vi "sub_conv_enc_v2.vi"(8 "code type":T1(ring)=enum."r=1/2 (13,17)", 11 "bitstream":i32[](array[numeric])) -> (3 "coded bits":i16[](array[numeric]))   [LabVIEW 2014]
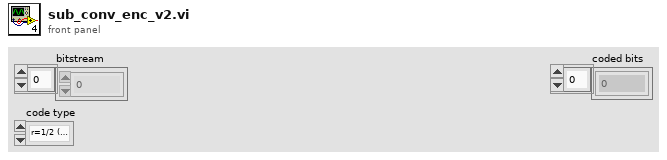
[diagram p1: front panel]
types:
  T1 = enum16{"r=1/2 (5,7)", "r=1/2 (13,17)", "r=1/4 (25,27,33,37)"}
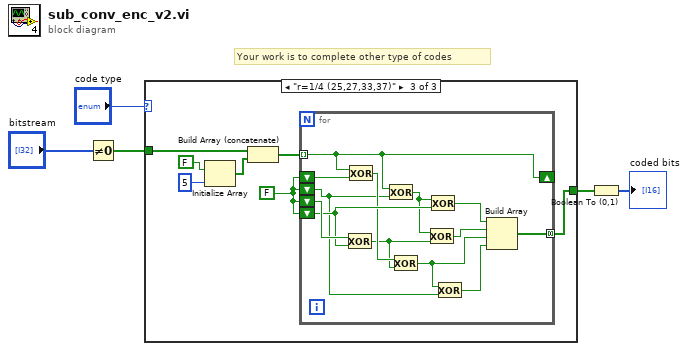
[diagram p0: block diagram]
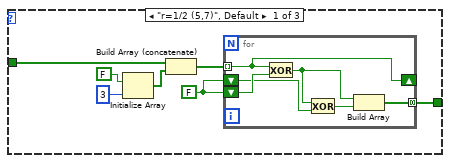
[diagram p2: hidden frame]
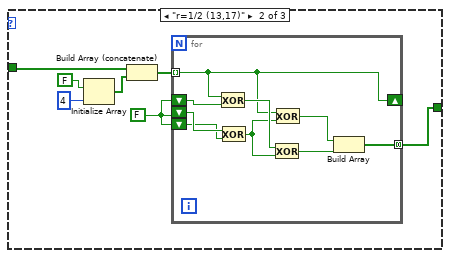
[diagram p3: hidden frame]
diagram:
  # "Your work is to complete other type of codes"
  n1 = Not Equal To 0?(x="bitstream") -> (x != 0?=w3:bool[])
  n2 = case shown="\"r=1/4 (25,27,33,37)\"" "code type" {
    tunnel: w3 -> [w8 w22 w38]
    tunnel: [w11 w20 w36] -> w2
    frame "r=1/2 (5,7)", Default {
      w12 = FALSE
      n3 = Initialize Array(FALSE, 3 ("dimension size")) -> (w7:bool[])
      n4 = Build Array (concatenate)(w8, w7) -> (w6:bool[])
      n5 = for {
        tunnel: w6 -> [w13] mode=indexing
        shift-right: [w13] -> _
        shift-left: w12 -> [w15]
        shift-left: w12 -> [w17]
        tunnel: [w18] -> w11 mode=concatenating
        n6 = Exclusive Or(1:w17, 2:w13) -> (0:w16:bool)
        n7 = Exclusive Or(1:w15, 2:w16) -> (0:w14:bool)
        n8 = Build Array(w16, w14) -> (w18:bool[])
      }
    }
    frame "r=1/2 (13,17)" {
      w19 = FALSE
      n9 = Initialize Array(FALSE, 4 ("dimension size")) -> (w23:bool[])
      n10 = Build Array (concatenate)(w22, w23) -> (w21:bool[])
      n11 = for {
        shift-right: [w29] -> _
        shift-left: w19 -> [w32]
        tunnel: w21 -> [w29] mode=indexing
        shift-left: w19 -> [w34]
        shift-left: w19 -> [w33]
        tunnel: [w26] -> w20 mode=concatenating
        n12 = Exclusive Or(1:w32, 2:w29) -> (0:w31:bool)
        n13 = Exclusive Or(1:w33, 2:w34) -> (0:w30:bool)
        n14 = Exclusive Or(1:w30, 2:w31) -> (0:w27:bool)
        n15 = Exclusive Or(1:w30, 2:w29) -> (0:w28:bool)
        n16 = Build Array(w28, w27) -> (w26:bool[])
      }
    }
    frame "r=1/4 (25,27,33,37)" {
      w35 = FALSE
      n17 = Initialize Array(FALSE, 5 ("dimension size")) -> (w39:bool[])
      n18 = Build Array (concatenate)(w38, w39) -> (w37:bool[])
      n19 = for {
        shift-right: [w53] -> _
        shift-left: w35 -> [w54]
        shift-left: w35 -> [w47]
        shift-left: w35 -> [w52]
        shift-left: w35 -> [w51]
        tunnel: w37 -> [w53] mode=indexing
        tunnel: [w42] -> w36 mode=concatenating
        n20 = Exclusive Or(1:w51, 2:w52) -> (0:w48:bool)
        n21 = Exclusive Or(1:w54, 2:w53) -> (0:w49:bool)
        n22 = Exclusive Or(1:w47, 2:w53) -> (0:w50:bool)
        n23 = Exclusive Or(1:w48, 2:w49) -> (0:w44:bool)
        n24 = Exclusive Or(1:w48, 2:w50) -> (0:w45:bool)
        n25 = Exclusive Or(1:w51, 2:w50) -> (0:w46:bool)
        n26 = Exclusive Or(1:w47, 2:w44) -> (0:w43:bool)
        n27 = Build Array(w46, w45, w44, w43) -> (w42:bool[])
      }
    }
  }
  n28 = Boolean To (0,1)(Boolean=w2) -> (0, 1=→"coded bits":i16[])
